vi "oax_Set Transition Pattern.vi"(10 "time period":dbl[](array[numeric]), 11 "speed":dbl[](array[numeric])) -> (1 "time period":dbl[](array[numeric]), 2 "end speed":dbl[](array[numeric]), 3 "start speed/constant speed":dbl[](array[numeric]))   [LabVIEW 2017]
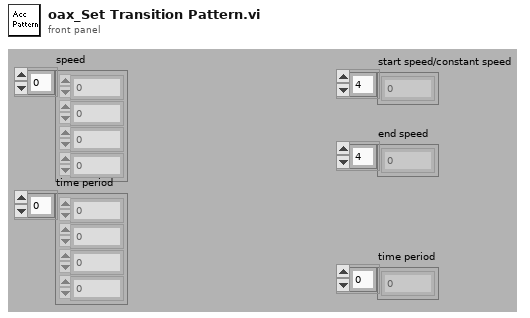
[diagram p1: front panel]
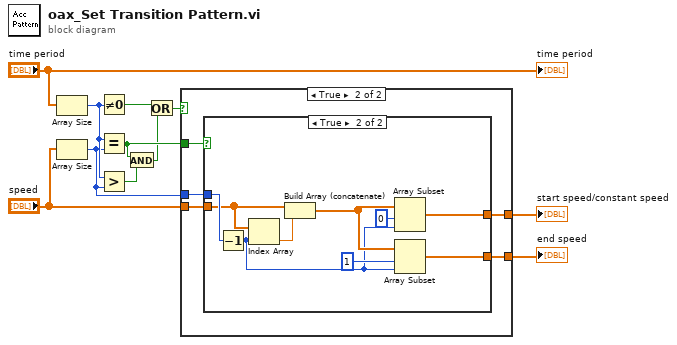
[diagram p0: block diagram]
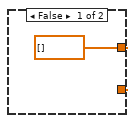
[diagram p2: hidden frame]
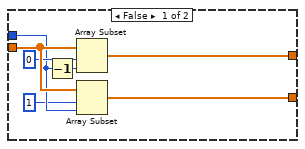
[diagram p3: hidden frame]
diagram:
  n1 = Array Size(array="time period") -> (size(s)=w8:i32)
  n2 = Array Size(array="speed") -> (size(s)=w3:i32)
  n3 = Not Equal To 0?(x=w8) -> (x != 0?=w10:bool)
  n4 = Equal?(x=w8, y=w3) -> (x = y?=w6:bool)
  n5 = Greater?(x=w8, y=w3) -> (0:w7:bool)
  n6 = And(x=w6, y=w7) -> (x .and. y?=w5:bool)
  n7 = Or(x=w10, y=w5) -> (x .or. y?=w9:bool)
  n8 = case shown="True" w9 {
    tunnel: w6 -> [_ w17]
    tunnel: "speed" -> [_ w16]
    tunnel: w3 -> [_ w15]
    tunnel: [w12 w14] -> w2
    tunnel: [w12 w13] -> w1
    frame False {
      w12 = dbl[] []
    }
    frame True {
      n9 = case shown="True" w17 {
        tunnel: w16 -> [w24 w29]
        tunnel: w15 -> [w21 w31]
        tunnel: [w19 w26] -> w14
        tunnel: [w18 w25] -> w13
        frame False {
          n10 = Decrement(x=w21) -> (x-1=w23:i32)
          n11 = Array Subset(array=w24, index=0, length=w23) -> (w19:dbl[])
          n12 = Array Subset(array=w24, index=1, length=w21) -> (w18:dbl[])
        }
        frame True {
          n13 = Decrement(x=w31) -> (x-1=w27:i32)
          n14 = Index Array(array=w29, index=w27) -> (element=w30:dbl)
          n15 = Build Array (concatenate)(w29, w30) -> (w28:dbl[])
          n16 = Array Subset(array=w28, index=0, length=w27) -> (w26:dbl[])
          n17 = Array Subset(array=w28, index=1, length=w27) -> (w25:dbl[])
        }
      }
    }
  }
  "start speed/constant speed" <- w2
  "end speed" <- w1
  "time period" <- "time period"
